vi "getSpeed_DriveQuadTalonSRX.vi"() -> (0 "Right Speed Ft/SEC":dbl format="%.4f", 3 "Left Speed FT/SEC":dbl format="%.4f")   [LabVIEW 2019, in "DriveQuadTalonSRX_Motor.lvlib"]
uses:
  DriveQuadTalonSRX_Motor.lvlib
  globals_DriveQuadTalonSRX.vi
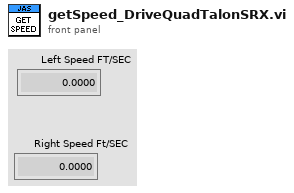
[diagram p1: front panel]
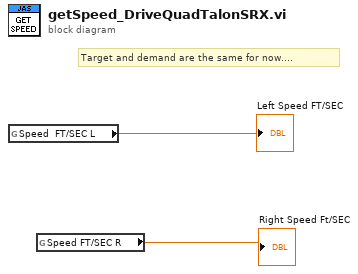
[diagram p0: block diagram]
diagram:
  # "Target and demand are the same for now...."
  n1 = global read "globals_DriveQuadTalonSRX.vi" "Speed  FT/SEC L"() -> (→"Left Speed FT/SEC":dbl)
  n2 = global read "globals_DriveQuadTalonSRX.vi" "Speed FT/SEC R"() -> (→"Right Speed Ft/SEC":dbl)
